vi "Process.vi"(8 "error in":errorcluster, 11 "Example Instrument UI":refnum<class "Instrument UI.PPMS.lvclass">) -> (0 "error out":errorcluster, 3 "Example Instrument UI out":refnum<class "Instrument UI.PPMS.lvclass">)   [LabVIEW 2019, in "Instrument UI.PPMS.lvclass"]
doc: "---------------------------------------------------------------\nJKI State Machine Objects™\nhttp://jki.net/state-machine-objects/\nCopyright (C) 2005-2015, JKI <info@jki.net>\nALL RIGHTS RESERVEDJKI State Machine Objects (SMO) 1.0.0.5\nJKI - JKI\nCopyright (c) 2016, JKI"
uses:
  Instrument UI.PPMS.lvclass
  <vilib>/JKI/JKI SMO/SMO/SMO.lvclass
  <vilib>/JKI/JKI SMO/SMO.UI/SMO.UI.lvclass
  <userlib>/LevyLab/Instrument Framework/Instrument/Instrument.lvclass
  instrument.PPMS/Typedefs/PPMS.getAll--cluster.ctl
  instrument.PPMS/instrument.PPMS.lvclass
  <vilib>/MakerHub/Toolbox/LMH-Toolbox.lvlib
  <userlib>/LevyLab/Instrument Framework/Instrument UI/Instrument UI.lvclass
  PPMS/PPMS.lvlib
  <userlib>/LevyLab/Configuration/Configuration.lvclass
  <userlib>/LevyLab/Instrument Framework/Instrument Types/Cryostat/Typedefs/Magnet Mode--Enum.ctl
  <userlib>/LevyLab/Instrument Framework/Instrument Types/Cryostat/Instrument.Cryostat.lvclass
  <userlib>/LevyLab/Instrument Framework/Instrument/Typedefs/Client Type--Enum.ctl
  63c30ead-59b5-487b-ba61-02a99048a75e.vi
  <userlib>/LevyLab/Instrument Framework/Instrument/API/Instrument.sendMessageToProcess (string).vi
  <userlib>/LevyLab/Debug/Debug.lvlib
  C:/Program Files (x86)/National Instruments/LabVIEW 2019/user.lib/LevyLab/Instrument Framework/Instrument UI/Instrument UI.lvclass
  C:/Program Files (x86)/National Instruments/LabVIEW 2019/vi.lib/JKI/JKI SMO/SMO.UI/SMO.UI.lvclass
  C:/Program Files (x86)/National Instruments/LabVIEW 2019/vi.lib/JKI/JKI SMO/SMO/SMO.lvclass
  C:/Program Files (x86)/National Instruments/LabVIEW 2019/user.lib/LevyLab/Instrument Framework/Instrument Types/Cryostat/Instrument.Cryostat.lvclass
  C:/Program Files (x86)/National Instruments/LabVIEW 2019/user.lib/LevyLab/Instrument Framework/Instrument/Instrument.lvclass
  instrument.PPMS/Typedefs/PPMS.Chamber Command--enum.ctl
panel:
  out "error":string="..."
  out "State":string="this is the text"
  in  "setChamber":bool
  in  "Chamber":T1="Seal"
  out "Chamber Status":string
  out "Angle (°)":dbl=90.0
  in  "setAngle":bool
  in  "Target Angle (°)":dbl format="%_3g"
  out "version":string
  out "Title":string="PPMSim"
  out "Time":dbl=90.002 format="%<%H:%M:%S %Y/%m/%d>T"
  in  "Mode":T2
  in  "B Rate (T/min)":dbl=0.1 format="%_3g"
  in  "T Rate (K/min)":dbl=300.0 format="%#_5g"
  in  "setField":bool
  in  "setTemperature":bool
  in  "Target Field (T)":dbl format="%_3g"
  in  "Target T (K)":dbl format="%#_5g"
  out "Temperature Status":string
  out "Magnet Status":string
  out "He Level (%)":dbl=90.0
  out "B (T)":dbl format="%_3f"
  out "T (K)":dbl=300.0 format="%#_5g"
  # "Local Targets"
  # "Status"
  # "SMO UI Template"
  # "For instructions on how to use the JKI State Machine Objects, examples and video tutorials, visit:\nhttp://jki.net/state-machine-objects/\n\nJKI State Machine Objects™\nhttp://jki.net/state-machine-objects/\nCopyright (C) 2005-2015, JKI <info@jki.net>\nALL RIGHTS RESERVED"
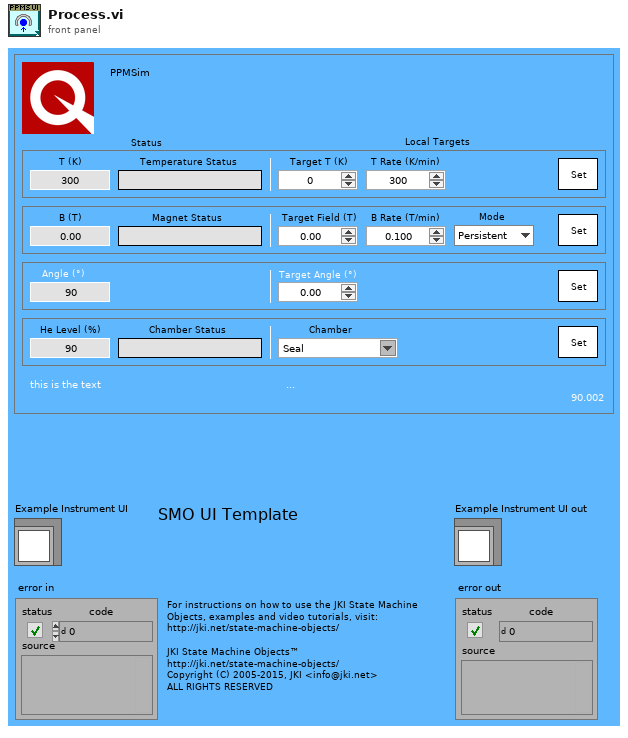
[diagram p1: front panel]
types:
  T1 = typedef "instrument.PPMS.lvclass/PPMS.Chamber Command--enum.ctl" = string
  T2 = typedef "Instrument.Cryostat.lvclass/Magnet Mode--Enum.ctl" = enum16{"Persistent", "Driven"}
  T3 = enum32{"invalid app kind", "Development System", "Run Time System", "Student Edition", "Embedded LabVIEW", "Evaluation", "Custom"}
  T4 = enum32{"Invalid", "Standard", "Closed", "Hidden", "Minimized", "Maximized"}
  T5 = typedef "instrument.PPMS.lvclass/PPMS.getAll--cluster.ctl" = cluster{"Chamber Status":string, "Helium Level":dbl, "Temperature":dbl, "Temperature Status":string, "Magnetic Field":dbl, "Magnet Status":string, "Position":dbl}
  T6 = typedef "Instrument.lvlib/Instrument.lvclass/Client Type--Enum.ctl" = enum16{"Remote", "Local"}
  T7 = typedef "PPMS.lvlib/Select PPMS--Enum.ctl" = enum16{"PPMS1", "PPMS2", "PPMS3", "PPMS-W-1", "OptiCool", "Simulate PPMS", "Simulate DynaCool", "Simulate OptiCool"}
  T8 = cluster{"Core":cluster{"Current VI Reference":refnum<vi>, "Close Panel on Exit?":bool, "Last Error":cluster{"error":errorcluster, "previous state":string, "remaining states":string}, "Shutdown?":bool}, "Instrument UI":refnum<class "Instrument UI.PPMS.lvclass">, "instrument.PPMS out":refnum<class "instrument.PPMS.lvclass">, "Data Send":variant, "Data Receive":variant, "getAll":T5, "UI Config":refnum<class "Configuration.lvclass">, "UI Cluster":cluster{"Target T (K)":dbl, "T Rate (K/min)":dbl, "Target Field (T)":dbl, "B Rate (T/min)":dbl, "Mode":T2, "Target Angle (°)":dbl}, "Client Type":T6, "Select PPMS":T7}
  T9 = cluster{"Current VI Reference":refnum<vi>, "Close Panel on Exit?":bool, "Last Error":cluster{"error":errorcluster, "previous state":string, "remaining states":string}, "Shutdown?":bool}
  T10 = cluster{"Target T (K)":dbl, "T Rate (K/min)":dbl, "Target Field (T)":dbl, "B Rate (T/min)":dbl, "Mode":T2, "Target Angle (°)":dbl}
  T11 = typedef "SMO.lvclass/Protected Events.ctl" = cluster{"StopProcesses":refnum<user-event>, "AbortProcesses":refnum<user-event>, "Config Changed":refnum<user-event>, "Dependency":refnum<user-event>}
  T12 = typedef "Instrument.lvlib/Instrument.lvclass/PublicEvents--Cluster.ctl" = cluster{"MessageFromProcess":refnum<user-event>}
  T13 = typedef "SMO.lvclass/Public Events.ctl" = cluster{"Error":refnum<user-event>, "State":refnum<user-event>, "Reserve State":refnum<user-event>}
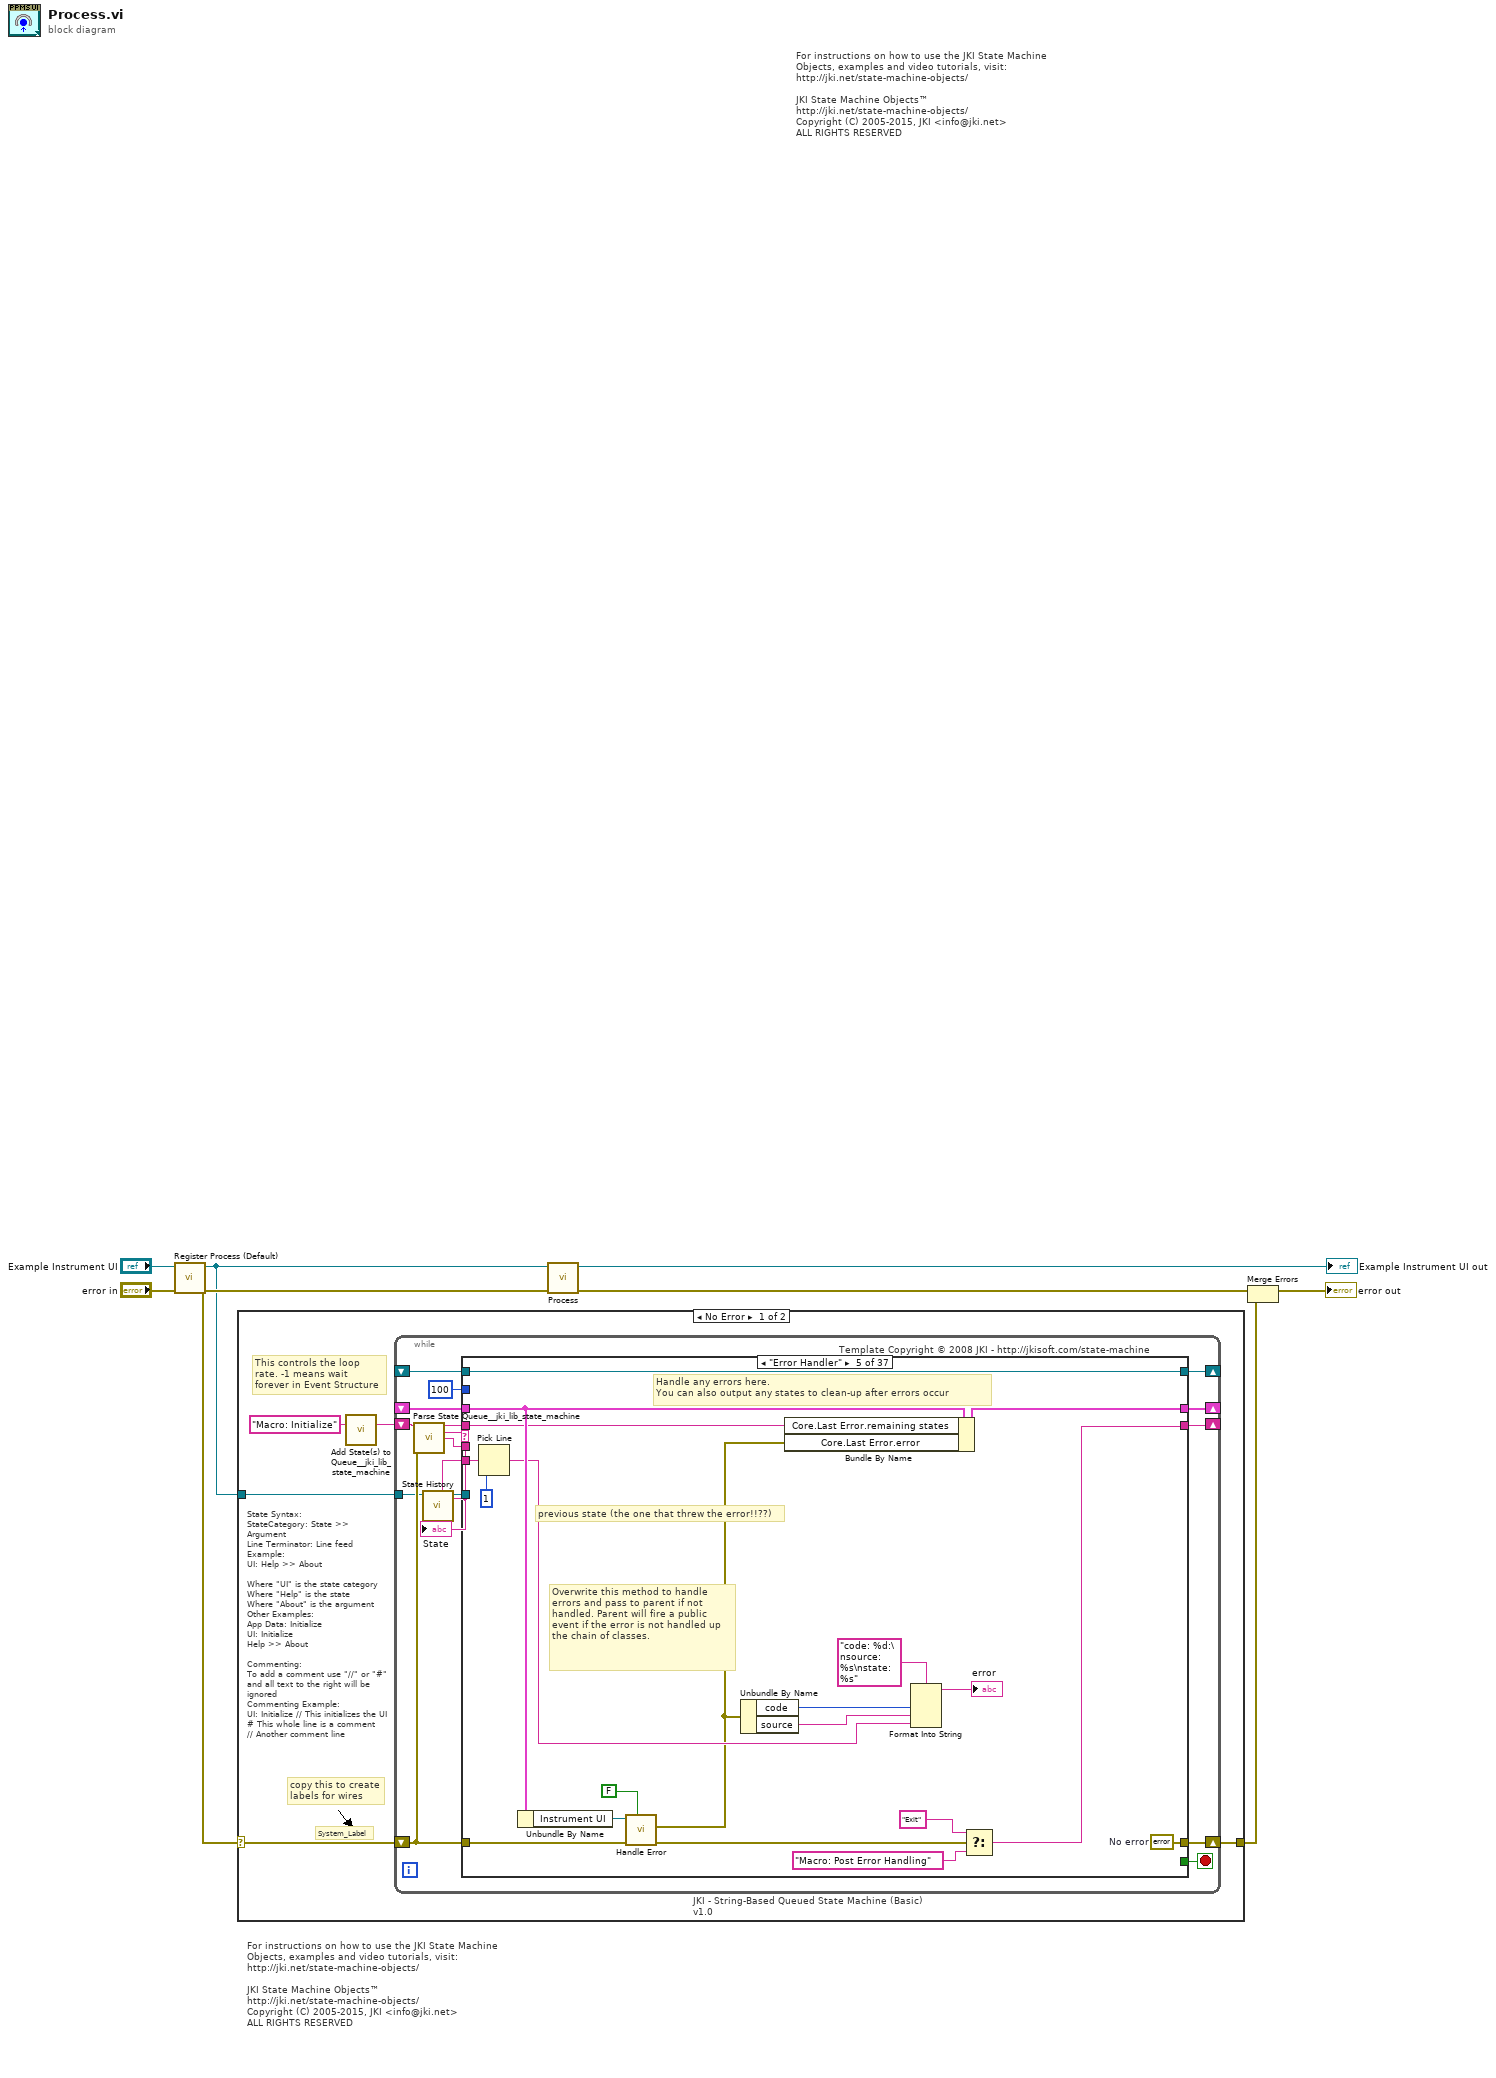
[diagram p0: block diagram]
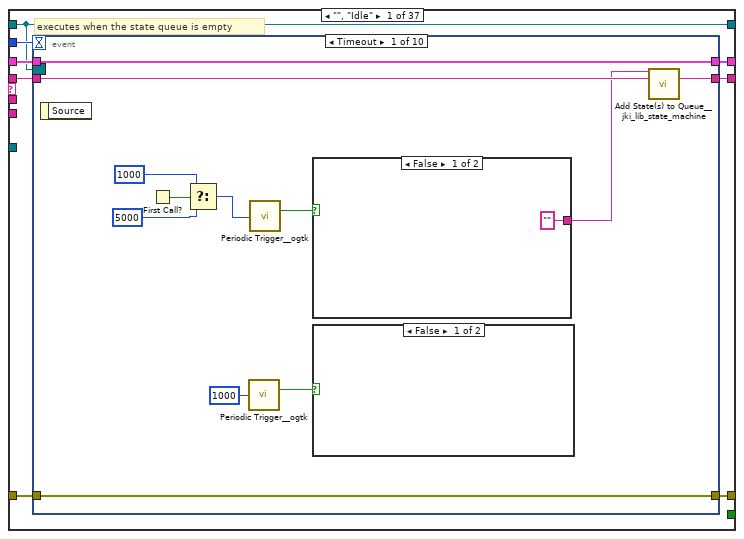
[diagram p2: hidden frame]
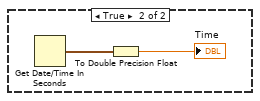
[diagram p3: hidden frame]
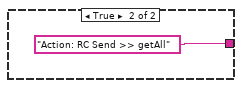
[diagram p4: hidden frame]
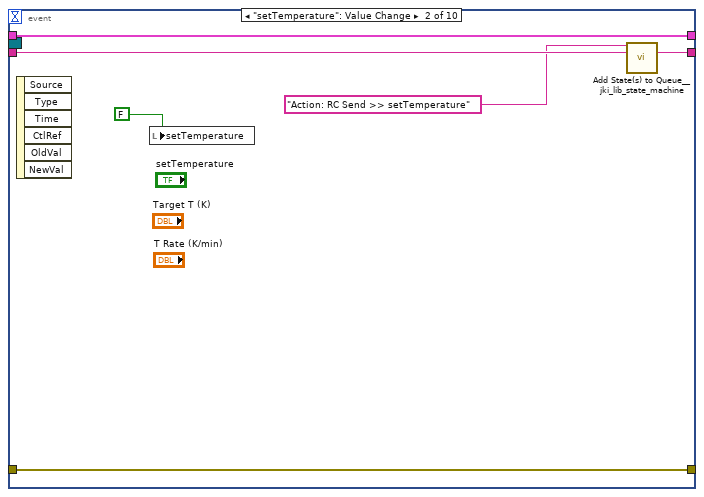
[diagram p5: hidden frame]
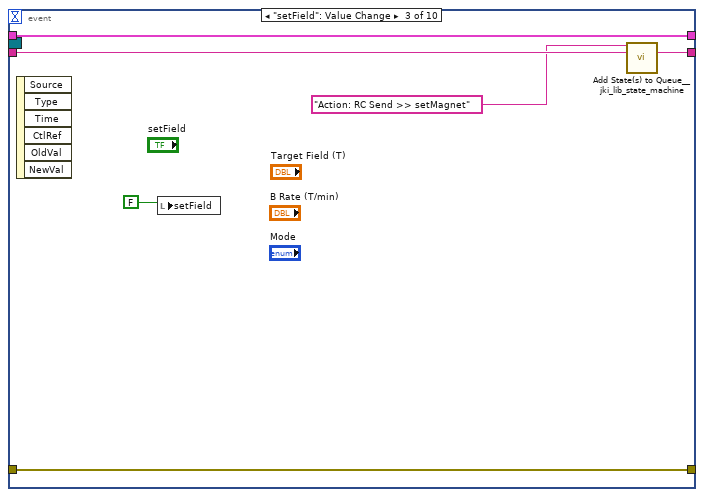
[diagram p6: hidden frame]
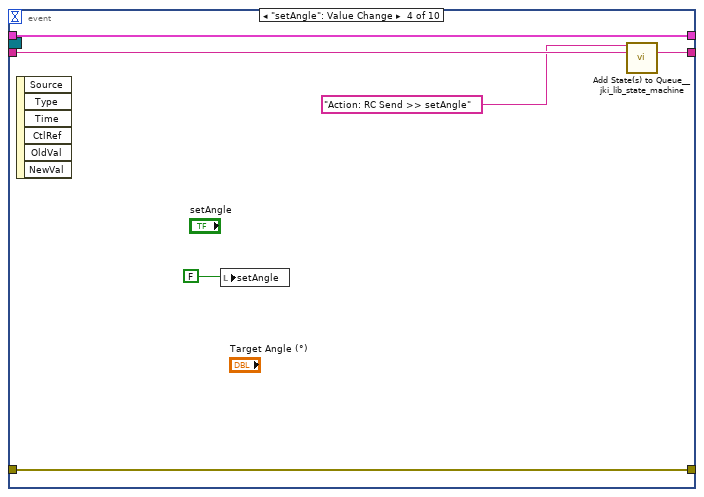
[diagram p7: hidden frame]
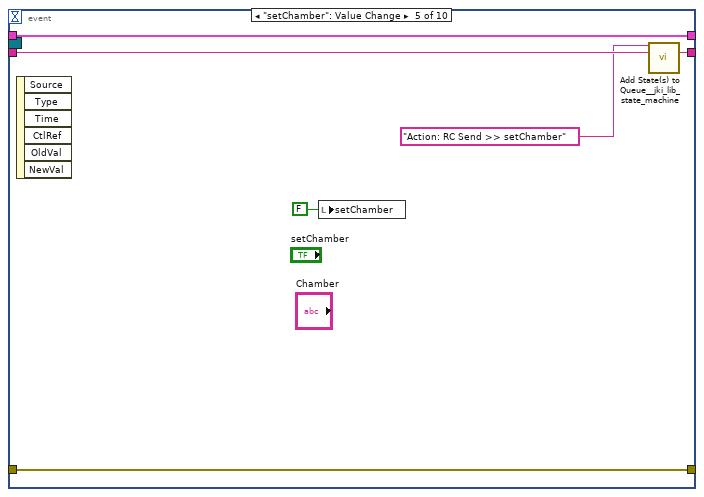
[diagram p8: hidden frame]
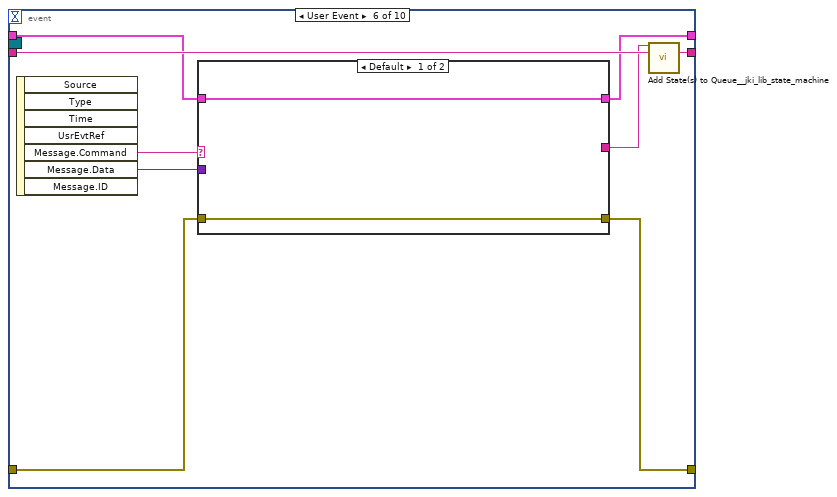
[diagram p9: hidden frame]
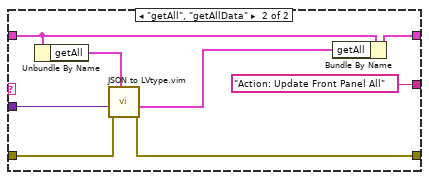
[diagram p10: hidden frame]
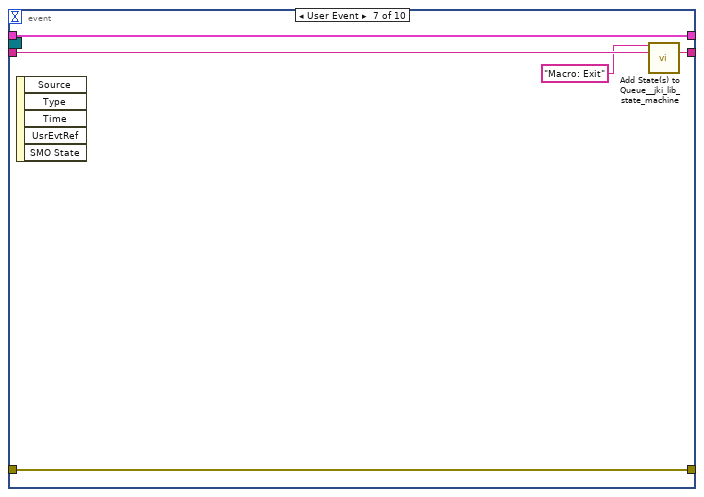
[diagram p11: hidden frame]
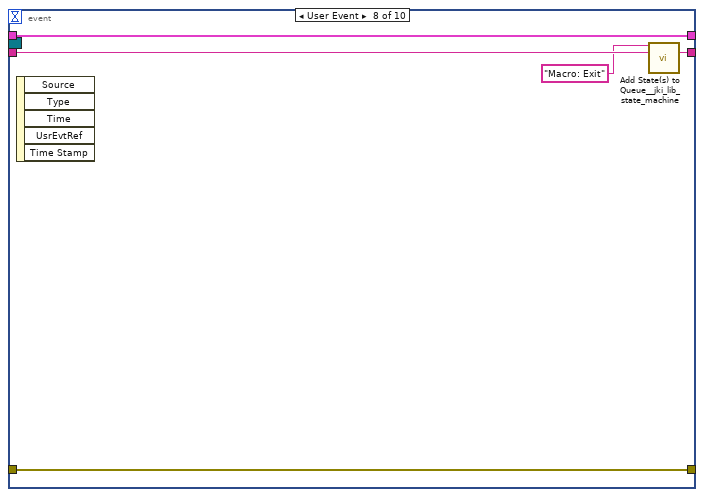
[diagram p12: hidden frame]
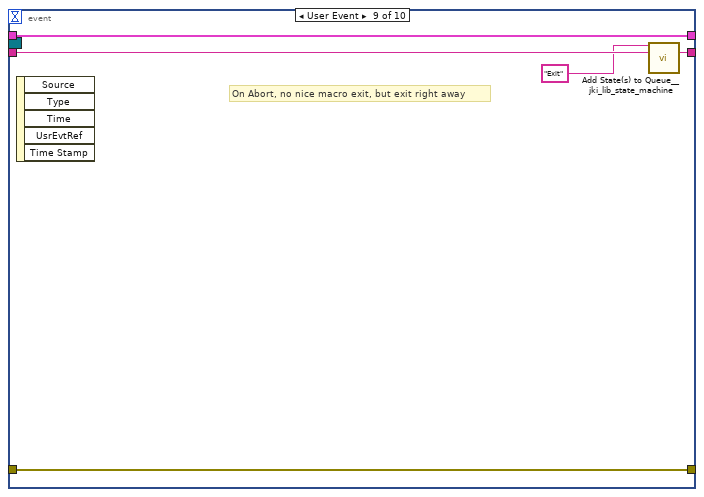
[diagram p13: hidden frame]
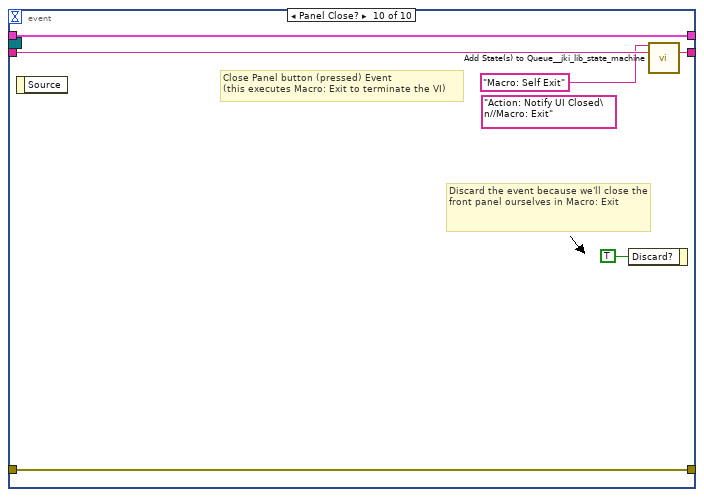
[diagram p14: hidden frame]
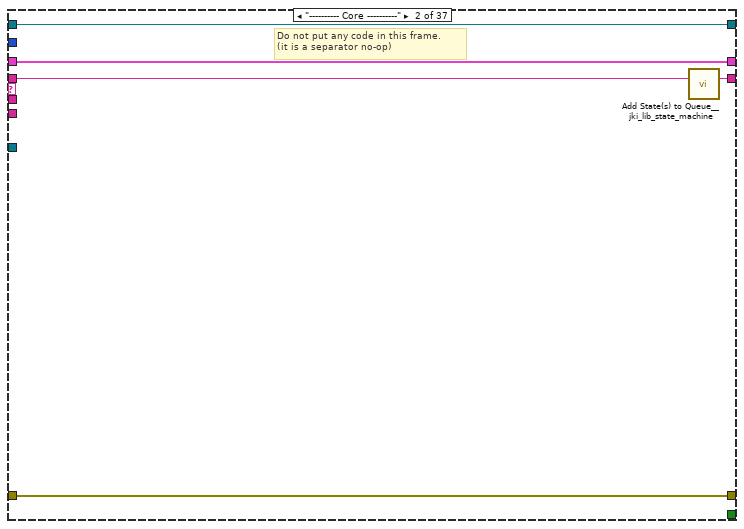
[diagram p15: hidden frame]
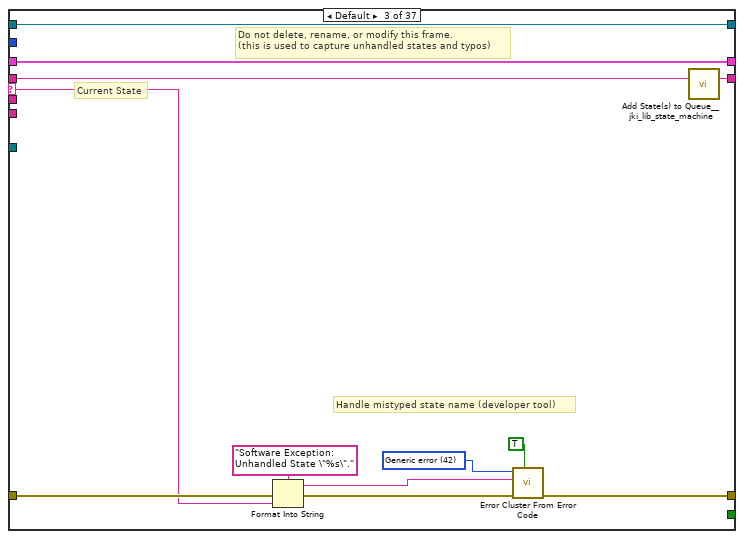
[diagram p16: hidden frame]
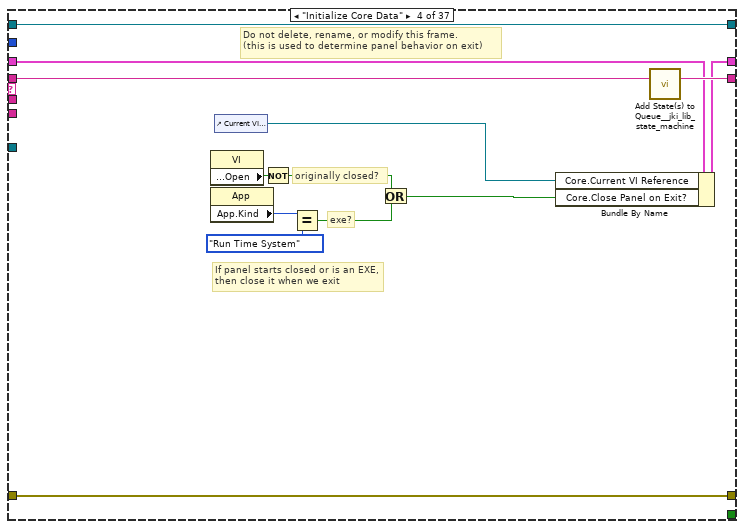
[diagram p17: hidden frame]
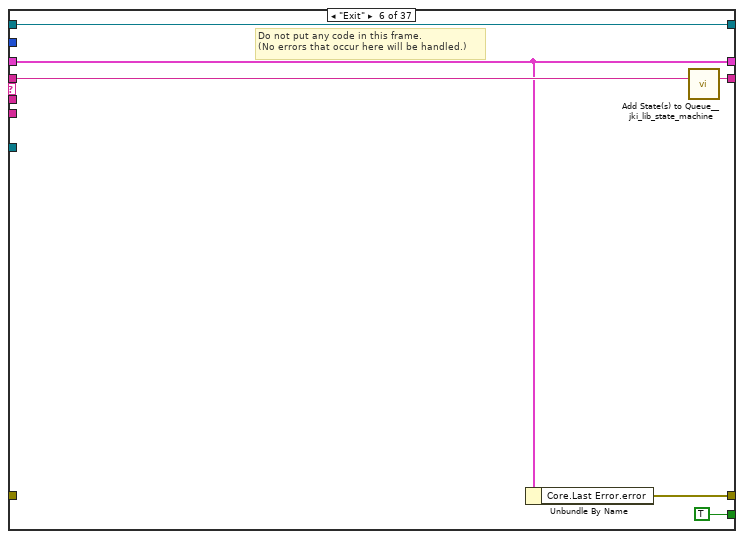
[diagram p18: hidden frame]
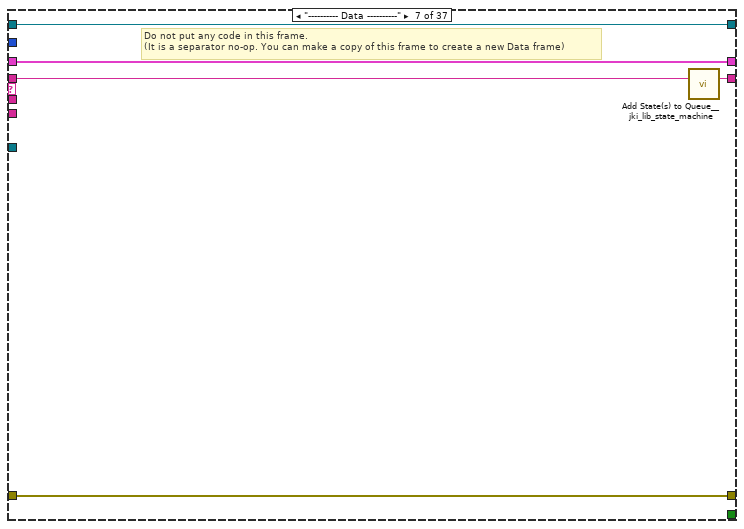
[diagram p19: hidden frame]
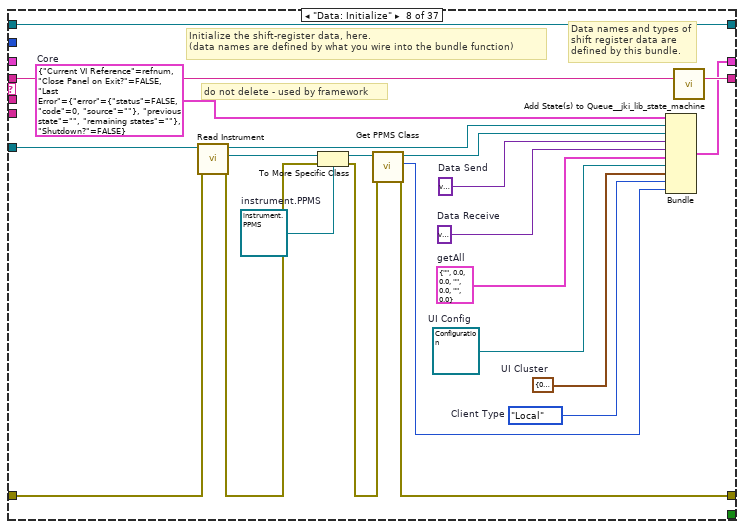
[diagram p20: hidden frame]
diagram:
  # "For instructions on how to use the JKI State Machine Objects, examples and video tutorials, visit:\nhttp://jki.net/state-machine-objects/\n\nJKI State Machine Objects™\nhttp://jki.net/state-machine-objects/\nCopyright (C) 2005-2015, JKI <info@jki.net>\nALL RIGHTS RESERVED"
  # "For instructions on how to use the JKI State Machine Objects, examples and video tutorials, visit:\nhttp://jki.net/state-machine-objects/\n\nJKI State Machine Objects™\nhttp://jki.net/state-machine-objects/\nCopyright (C) 2005-2015, JKI <info@jki.net>\nALL RIGHTS RESERVED"
  n1 = call <vilib>:"Register Process (Default).vi"("error in (no error)"="error in", "SMO"="Example Instrument UI") -> ("error out"=w5:errorcluster, "SelfRef"=w4:refnum<class "Instrument UI.PPMS.lvclass">)  [unwired: 8 in]
  n2 = case shown="No Error" w5 {
    selector: w5 -> [w10 w589]
    tunnel: w4 -> [w11 _]
    tunnel: [w9 w589] -> w1
    frame No Error {
      # "State Syntax:\nStateCategory: State >> Argument\nLine Terminator: Line feed\nExample:\nUI: Help >> About\n\nWhere \"UI\" is the state category\nWhere \"Help\" is the state\nWhere \"About\" is the argument\nOther Examples:\nApp Data: Initialize\nUI: Initialize\nHelp >> About\n\nCommenting:\nTo add a comment use \"//\" or \"#\" and all text to the right will be ignored\nCommenting Example:\nUI: Initialize // This initializes the UI\n# This whole line is a comment\n// Another comment line"
      # "copy this to create labels for wires"
      # "This controls the loop rate. -1 means wait forever in Event Structure"
      # "System_Label"
      n3 = call <vilib>:"Add State(s) to Queue__jki_lib_state_machine.vi"("State(s) in (\"\")"="Macro: Initialize") -> ("States Out"=w13:string)  [unwired: 14 in]
      n4 = while "JKI - String-Based Queued State Machine (Basic) v1.0" {
        shift-right: [w24] -> _
        shift-left: _ -> [w23]
        shift-right: [w18] -> w9
        shift-left: w10 -> [w21]
        shift-right: [w26] -> _
        shift-left: w13 -> [w27]
        tunnel: w11 -> [w16]
        shift-right: [w20] -> _
        shift-left: _ -> [w19]
        stop <- w25 stop-if-true
        # "Template Copyright © 2008 JKI - http://jkisoft.com/state-machine"
        n5 = call <vilib>:"Parse State Queue__jki_lib_state_machine.vi"("State Queue"=w27, "Error In (no error)"=w21) -> ("Remaining States"=w29:string, "Current State"=w15:string, "Arguments"=w28:string)  [unwired: 11 in]
        "State" <- w15
        n6 = call <userlib>:"State History.vi"("Current State"=w15, "SMO"=w16) -> ("SMO"=w17:refnum<class "Instrument UI.PPMS.lvclass">, "History"=w14:string)  [unwired: 8 in]
        n7 = case shown="\"Error Handler\"" w15 {
          selector: w15 -> [_ _ w124 _ _ _ _ _ _ _ _ _ _ _ _ _ _ _ _ _ _ _ _ _ _ _ _ _ _ _ _ _ _ _ _ _ _]
          tunnel: w29 -> [w37 w122 w128 w147 w149 w173 w178 w200 w208 w213 w220 w227 w243 w285 w305 w330 w354 w371 w390 w395 w404 w414 _ w446 w451 w462 w469 w476 w481 w497 w503 w510 w517 w530 w540 w547 w558]
          tunnel: w28 -> [_ _ _ _ _ _ _ _ _ _ _ w221 w237 _ _ _ _ _ _ _ _ _ _ _ _ _ _ _ _ _ _ _ _ _ _ _ w552]
          tunnel: w23 -> [w35 w119 w126 w138 w161 w169 w175 _ w205 w210 w218 w225 w239 w274 w295 w326 w350 w367 w386 w392 w400 w411 w416 w430 w448 w459 w464 w473 w478 w495 w501 w504 w511 w522 w537 w544 w548]
          tunnel: w21 -> [w33 w120 w129 w144 w162 _ w176 w184 w202 w211 w216 w223 w241 w271 w301 w324 w348 w365 w383 w393 w402 w412 w424 w444 w449 w454 w466 w472 w479 w492 w499 w507 w513 w524 w531 w541 w553]
          tunnel: [w36 w121 w127 w146 w150 w172 w177 w199 w207 w212 w219 w226 w242 w284 w304 w329 w353 w370 w389 w394 w403 w413 w425 w445 w450 w461 w468 w475 w480 w496 w502 w509 w516 w529 w539 w546 w557] -> w26
          tunnel: [_ _ _ _ _ TRUE _ _ _ _ _ _ _ _ _ _ _ _ _ _ _ _ _ _ _ _ _ _ _ _ _ _ _ _ _ _ _] -> w25
          tunnel: [w32 w119 w126 w145 w164 w169 w175 w198 w205 w210 w218 w225 w239 w275 w296 w327 w351 w368 w387 w392 w400 w411 w417 w431 w448 w459 w464 w473 w478 w495 w501 w506 w511 w522 w536 w543 w549] -> w24
          tunnel: 100 ("Timeout") -> [w31 _ _ _ _ _ _ _ _ _ _ _ _ _ _ _ _ _ _ _ _ _ _ _ _ _ _ _ _ _ _ _ _ _ _ _ _]
          tunnel: w17 -> [_ _ _ _ _ _ _ w186 _ _ _ _ _ _ _ _ _ _ _ _ _ _ _ _ _ _ _ _ _ _ _ _ _ _ _ _ _]
          tunnel: [w30 w118 w123 w135 w167 w170 w174 w197 w204 w209 w217 w224 w236 w283 w303 w328 w352 w369 w388 w391 w401 w410 w423 w438 w447 w460 w467 w474 w477 w494 w500 w508 w515 w528 w538 w545 w556] -> w20
          tunnel: w19 -> [w30 w118 w123 w135 w167 w170 w174 w197 w204 w209 w217 w224 w236 w283 w303 w328 w352 w369 w388 w391 w401 w410 w423 w438 w447 w460 w467 w474 w477 _ w500 w508 w515 w528 w538 w545 w556]
          tunnel: [w34 w120 w130 w144 w165 w168 w176 w179 w206 w211 w215 w222 w240 w271 w301 w324 w342 w364 w382 w393 w402 w412 w424 w444 w449 w453 w465 w471 w479 w490 w498 w507 w512 w524 w532 w541 w554] -> w18
          tunnel: w14 -> [_ _ _ _ w155 _ _ _ _ _ _ _ _ _ _ _ _ _ _ _ _ _ _ _ _ _ _ _ _ _ _ _ _ _ _ _ _]
          frame "", "Idle" {
            # "executes when the state queue is empty"
            n8 = event shown="[0] Timeout" {
              selector: w30 -> [_ _ _ _ _ _ _ _ _ _]
              dyn-events: _ -> [_ _ _ _ _ _ _ _ _ _]
              timeout: w31 -> [_ _ _ _ _ _ _ _ _ _]
              tunnel: w37 -> [w49 w56 w62 w68 w77 w86 w101 w106 w111 w117]
              tunnel: [w48 w58 w64 w70 w76 w85 w100 w105 w110 w116] -> w36
              tunnel: w35 -> [w46 w57 w63 w69 w74 w80 w98 w103 w108 w114]
              tunnel: [w47 w59 w65 w71 w75 w78 w99 w104 w109 w113] -> w34
              tunnel: w33 -> [w47 w59 w65 w71 w75 w79 w99 w104 w109 w113]
              tunnel: [w46 w57 w63 w69 w74 w81 w98 w103 w108 w114] -> w32
              event Timeout {
                n9 = event-data() -> ()  [unwired: 1 in, 1 out]
                n10 = First Call?() -> (First Call?: T/F=w41:bool)
                n11 = Select(t=u32 1000 ("update time (ms)"), s=w41, f=u32 5000 ("update time (ms)")) -> (s? t:f=w38:u32)
                n12 = call <userlib>:"Periodic Trigger__ogtk.vi"("time (ms)"=u32 1000) -> ("Triggered"=w42:bool)  [unwired: 12 in, 2 out]
                n13 = call <userlib>:"Periodic Trigger__ogtk.vi"("time (ms)"=w38) -> ("Triggered"=w45:bool)  [unwired: 12 in, 2 out]
                n14 = case shown="False" w45 {
                  tunnel: ["" "Action: RC Send >> getAll"] -> w44
                  frame False {
                  }
                  frame True {
                  }
                }
                n15 = case shown="False" w42 {
                  frame False {
                  }
                  frame True {
                    n16 = Get Date/Time In Seconds() -> (seconds since 1Jan1904=w51:timestamp)
                    n17 = To Double Precision Float(number=w51) -> (double precision float=→"Time":dbl)
                  }
                }
                n18 = call <vilib>:"Add State(s) to Queue__jki_lib_state_machine.vi"("State(s) in Front (\"\")"=w44, "State(s) in (\"\")"=w49) -> ("States Out"=w48:string)  [unwired: 13 in]
              }
              event "setTemperature": Value Change {
                n19 = event-data() -> ()  [unwired: 1 in, 6 out]
                n20 = local write "setTemperature"(FALSE ("Temperature")) -> ()
                n21 = call <vilib>:"Add State(s) to Queue__jki_lib_state_machine.vi"("State(s) in Front (\"\")"="Action: RC Send >> setTemperature" ("State(s) in Front (\"\")"), "State(s) in (\"\")"=w56) -> ("States Out"=w58:string)  [unwired: 13 in]
              }
              event "setField": Value Change {
                n22 = event-data() -> ()  [unwired: 1 in, 6 out]
                n23 = local write "setField"(FALSE ("Field")) -> ()
                n24 = call <vilib>:"Add State(s) to Queue__jki_lib_state_machine.vi"("State(s) in Front (\"\")"="Action: RC Send >> setMagnet" ("State(s) in Front (\"\")"), "State(s) in (\"\")"=w62) -> ("States Out"=w64:string)  [unwired: 13 in]
              }
              event "setAngle": Value Change {
                n25 = event-data() -> ()  [unwired: 1 in, 6 out]
                n26 = local write "setAngle"(FALSE ("Angle")) -> ()
                n27 = call <vilib>:"Add State(s) to Queue__jki_lib_state_machine.vi"("State(s) in Front (\"\")"="Action: RC Send >> setAngle" ("State(s) in Front (\"\")"), "State(s) in (\"\")"=w68) -> ("States Out"=w70:string)  [unwired: 13 in]
              }
              event "setChamber": Value Change {
                n28 = event-data() -> ()  [unwired: 1 in, 6 out]
                n29 = local write "setChamber"(FALSE ("Set Chamber")) -> ()
                n30 = call <vilib>:"Add State(s) to Queue__jki_lib_state_machine.vi"("State(s) in Front (\"\")"="Action: RC Send >> setChamber" ("State(s) in Front (\"\")"), "State(s) in (\"\")"=w77) -> ("States Out"=w76:string)  [unwired: 13 in]
              }
              event User Event {
                n31 = event-data() -> ("Message.Command"=w83:string, "Message.Data"=w82:variant)  [unwired: 1 in, 5 out]
                n32 = case shown="Default" w83 {
                  tunnel: [_ "Action: Update Front Panel All" ("State(s) in Front (\"\")")] -> w84
                  tunnel: w82 -> [_ w94]
                  tunnel: w80 -> [w88 w89]
                  tunnel: [w88 w95] -> w81
                  tunnel: w79 -> [w87 w90]
                  tunnel: [w87 w91] -> w78
                  frame Default {
                  }
                  frame "getAll", "getAllData" {
                    n33 = Unbundle By Name(w89) -> ("getAll"=w93:T5)
                    n34 = call "JSON to LVtype.vim"("type"=w93, "error in (no error)"=w90, "JSON Data in"=w94) -> ("error out"=w91:errorcluster, "Data out"=w92:T5)  [unwired: 7 in]
                    n35 = Bundle By Name(cluster=w89, "getAll"=w92) -> (w95:T8)
                  }
                }
                n36 = call <vilib>:"Add State(s) to Queue__jki_lib_state_machine.vi"("State(s) in Front (\"\")"=w84, "State(s) in (\"\")"=w86) -> ("States Out"=w85:string)  [unwired: 13 in]
              }
              event User Event {
                n37 = event-data() -> ()  [unwired: 1 in, 5 out]
                n38 = call <vilib>:"Add State(s) to Queue__jki_lib_state_machine.vi"("State(s) in Front (\"\")"="Macro: Exit", "State(s) in (\"\")"=w101) -> ("States Out"=w100:string)  [unwired: 13 in]
              }
              event User Event {
                n39 = event-data() -> ()  [unwired: 1 in, 5 out]
                n40 = call <vilib>:"Add State(s) to Queue__jki_lib_state_machine.vi"("State(s) in Front (\"\")"="Macro: Exit", "State(s) in (\"\")"=w106) -> ("States Out"=w105:string)  [unwired: 13 in]
              }
              event User Event {
                # "On Abort, no nice macro exit, but exit right away"
                n41 = event-data() -> ()  [unwired: 1 in, 5 out]
                n42 = call <vilib>:"Add State(s) to Queue__jki_lib_state_machine.vi"("State(s) in Front (\"\")"="Exit", "State(s) in (\"\")"=w111) -> ("States Out"=w110:string)  [unwired: 13 in]
              }
              event Panel Close? {
                (unwired) "Action: Notify UI Closed\n//Macro: Exit"
                # "Discard the event because we'll close the front panel ourselves in Macro: Exit"
                # "Close Panel button (pressed) Event\n(this executes Macro: Exit to terminate the VI)"
                n43 = event-data() -> ()  [unwired: 1 in, 1 out]
                n44 = event-data("Discard?"=TRUE) -> ()  [unwired: 1 in, 1 out]
                n45 = call <vilib>:"Add State(s) to Queue__jki_lib_state_machine.vi"("State(s) in Front (\"\")"="Macro: Self Exit" ("State(s) in Front (\"\")"), "State(s) in (\"\")"=w117) -> ("States Out"=w116:string)  [unwired: 13 in]
              }
            }
          }
          frame "---------- Core ----------" {
            # "Do not put any code in this frame.\n(it is a separator no-op)"
            n46 = call <vilib>:"Add State(s) to Queue__jki_lib_state_machine.vi"("State(s) in (\"\")"=w122) -> ("States Out"=w121:string)  [unwired: 14 in]
          }
          frame Default {
            w133 = 42 items=["No error", "Argument error", "Memory is full", "Out of zone", "End of file", "File already open", "Generic file I/O error", "File not found", "File permission error", "Disk is full", "Duplicate path", "Too many files open", "System feature not enabled", "Resource file not found", "Cannot add resource", "Resource not found", "Image not found", "Image memory error", "Pen does not exist", "Config type invalid", "Config token not found", "Config parse error", "Config memory error", "Bad external code format", "Bad external code offset", "External code not present", "Null window", "Destroy window error", "Null menu", "Print aborted", "Bad print record", "Print driver error", "Windows error during printing", "Memory error during printing", "Print dialog error", "Generic print error", "Invalid device refnum", "Device not found", "Device parameter error", "Device unit error", "Cannot open device", "Device call aborted", "Generic error", "Cancelled by user", "Object ID too low", "Object ID too high", "Object not in heap", "Unknown heap", "Unknown object (invalid DefProc)", "Unknown object (DefProc not in table)", "Message out of range", "Invalid (null) method", "Unknown message", "Manager call not supported", "Bad address", "Network operation in progress", "Network operation timed out", "Connection is busy", "Network attribute not supported", "Network error", "Address in use", "System out of memory", "Connection aborted", "Connection refused", "Not connected", "Already connected", "Connection closed", "Initialization error (interapplication manager)", "Bad occurrence", "Wait on unbound occurrence handler", "Occurrence queue overflow", "Datalog type conflict", "Unused", "Unrecognized type (interapplication manager)", "Memory corrupt", "Failed to make temporary DLL", "Old CIN version", "Drag socket not found", "Failed to load drop-object", "Failed to register OLE object", "Failed to release OLE object", "Format specifier type mismatch", "Unknown format specifier", "Too few format specifiers", "Too many format specifiers", "Scan failed", "Newer CIN version", "Error converting to variant", "Runtime menu error", "Password tampered", "Variant attribute not found", "Incompatible variant data type", "Event data is not available", "Event Store is not present", "Occurrence is not found", "Event Queue is not created", "Event info is not available", "Refnum passed is NULL", "Error retrieving Class GUID", "Error retrieving CoClass GUID", "Error retrieving TypeLib GUID.", "Bad built application magic bytes.", "Specific driver is different from the specific driver associated with the Logical Name.", "There is no session opened to the class driver.", "Max Error", "MAX - Error with config objects", "MAX - Error loading configuration", "MAX - Group not supported"]
            # "Current State"
            # "Do not delete, rename, or modify this frame.\n(this is used to capture unhandled states and typos)"
            # "Handle mistyped state name (developer tool)"
            n47 = Format Into String(format string="Software Exception: Unhandled State \"%s\"." ("message"), error in=w129, w124) -> (resulting string=w132:string, error out=w131:errorcluster)  [unwired: 1 in]
            n48 = call <vilib>:"Error Cluster From Error Code.vi"("show call chain? (False)"=TRUE, "error in (no error)"=w131, "error message (\"\")"=w132, "error code (0)"=w133) -> ("error out"=w130:errorcluster)  [unwired: 5 in]
            n49 = call <vilib>:"Add State(s) to Queue__jki_lib_state_machine.vi"("State(s) in (\"\")"=w128) -> ("States Out"=w127:string)  [unwired: 14 in]
          }
          frame "Initialize Core Data" {
            # "Do not delete, rename, or modify this frame.\n(this is used to determine panel behavior on exit)"
            # "originally closed?"
            # "exe?"
            # "If panel starts closed or is an EXE, then close it when we exit"
            n50 = property class="VI"() -> ("Front Panel.Open"=w143:bool)  [unwired: 2 in, 2 out]
            n51 = property class="App"() -> ("App.Kind"=w142:T3)  [unwired: 2 in, 2 out]
            n52 = control-ref of="Current VI Reference"() -> (w136:refnum<vi>)
            n53 = Not(x=w143) -> (.not. x?=w140:bool)
            n54 = Equal?(x=w142, y=T3."Run Time System" ("Application:Kind")) -> (x = y?=w139:bool)
            n55 = Or(x=w140, y=w139) -> (x .or. y?=w137:bool)
            n56 = Bundle By Name(cluster=w138, "Core.Current VI Reference"=w136, "Core.Close Panel on Exit?"=w137) -> (w145:T8)
            n57 = call <vilib>:"Add State(s) to Queue__jki_lib_state_machine.vi"("State(s) in (\"\")"=w147) -> ("States Out"=w146:string)  [unwired: 14 in]
          }
          frame "Error Handler" {
            w165 = errorcluster {"status"=FALSE, "code"=0, "source"=""}  # No error
            # "previous state (the one that threw the error!!??)"
            # "Overwrite this method to handle errors and pass to parent if not handled. Parent will fire a public event if the error is not handled up the chain of classes."
            # "Handle any errors here.\nYou can also output any states to clean-up after errors occur"
            n58 = Pick Line(multi-line string=w155, line index=1) -> (output string=w153:string)  [unwired: 1 in]
            n59 = Unbundle By Name(w161) -> ("Instrument UI"=w166:refnum<class "Instrument UI.PPMS.lvclass">)
            n60 = call-dynamic "Handle Error.vi"("Stop on Unhandled Error (T)"=FALSE, "error in"=w162, "SMO"=w166) -> ("handling error"=w160:errorcluster, "Unhandled error"=w148:errorcluster)  [unwired: 6 in, 1 out]
            n61 = Unbundle By Name(w148) -> ("code"=w157:i32, "source"=w156:string)
            n62 = Bundle By Name(cluster=w161, "Core.Last Error.remaining states"=w149, "Core.Last Error.error"=w148) -> (w164:T8)
            n63 = Format Into String(format string="code: %d:\nsource: %s\nstate: %s", w157, w156, w153) -> (resulting string=→"error":string)  [unwired: 2 in, 1 out]
            n64 = Select(t="Exit", s=w160, f="Macro: Post Error Handling") -> (s? t:f=w150:string)
          }
          frame "Exit" {
            # "Do not put any code in this frame.\n(No errors that occur here will be handled.)"
            n65 = Unbundle By Name(w169) -> ("Core.Last Error.error"=w168:errorcluster)
            n66 = call <vilib>:"Add State(s) to Queue__jki_lib_state_machine.vi"("State(s) in (\"\")"=w173) -> ("States Out"=w172:string)  [unwired: 14 in]
          }
          frame "---------- Data ----------" {
            # "Do not put any code in this frame.\n(It is a separator no-op. You can make a copy of this frame to create a new Data frame)"
            n67 = call <vilib>:"Add State(s) to Queue__jki_lib_state_machine.vi"("State(s) in (\"\")"=w178) -> ("States Out"=w177:string)  [unwired: 14 in]
          }
          frame "Data: Initialize" {
            w185 = T9 {"Current VI Reference"=refnum, "Close Panel on Exit?"=FALSE, "Last Error"={"error"={"status"=FALSE, "code"=0, "source"=""}, "previous state"="", "remaining states"=""}, "Shutdown?"=FALSE}  # Core
            w187 = Client_Type--Enum."Local"  # Client Type
            w188 = T10 {"Target T (K)"=0.0, "T Rate (K/min)"=0.0, "Target Field (T)"=0.0, "B Rate (T/min)"=0.0, "Mode"=enum."Persistent", "Target Angle (°)"=0.0}  # UI Cluster
            w189 = refnum<class "Configuration.lvclass"> refnum  # UI Config
            w190 = refnum<class "instrument.PPMS.lvclass"> refnum  # instrument.PPMS
            w194 = T5 {"Chamber Status"="", "Helium Level"=0.0, "Temperature"=0.0, "Temperature Status"="", "Magnetic Field"=0.0, "Magnet Status"="", "Position"=0.0}  # getAll
            w195 = variant  # Data Receive
            w196 = variant  # Data Send
            # "do not delete - used by framework"
            # "Data names and types of shift register data are defined by this bundle."
            # "Initialize the shift-register data, here.\n(data names are defined by what you wire into the bundle function)"
            n68 = call <userlib>:"Read Instrument.vi"("error in (no error)"=w184, "Instrument UI in"=w186) -> ("error out"=w193:errorcluster, "Instrument"=w191:refnum<class "Instrument.lvclass">, "Instrument UI"=w192:refnum<class "Instrument UI.PPMS.lvclass">)  [unwired: 7 in]
            n69 = To More Specific Class(target class=w190, reference=w191, error in=w193) -> (specific class reference=w182:refnum<class "instrument.PPMS.lvclass">, error out=w180:errorcluster)
            n70 = call "Get PPMS Class.vi"("error in (no error)"=w180, "instrument.PPMS"=w182) -> ("error out"=w179:errorcluster, "Select PPMS"=w183:T7, "instrument.PPMS out"=w181:refnum<class "instrument.PPMS.lvclass">)  [unwired: 7 in]
            n71 = Bundle("Core"=w185, "Instrument UI"=w192, "instrument.PPMS out"=w181, "Data Send"=w196, "Data Receive"=w195, "getAll"=w194, "UI Config"=w189, "UI Cluster"=w188, "Client Type"=w187, "Select PPMS"=w183) -> (w198:T8)  [unwired: 1 in]
            n72 = call <vilib>:"Add State(s) to Queue__jki_lib_state_machine.vi"("State(s) in (\"\")"=w200) -> ("States Out"=w199:string)  [unwired: 14 in]
          }
          frame "Data: Cleanup" {
            # "Cleanup any data and references, here.\n(this is called automatically, by the Macro: Exit)"
            n73 = Unbundle By Name(w205) -> ("Core.Current VI Reference"=w203:refnum<vi>)
            n74 = call <vilib>:"Save State As Default.vi"("Error In"=w202, "Target VI"=w203) -> ("Error Out"=w201:errorcluster)  [unwired: 8 in, 1 out]
            n75 = Close Reference(reference=w203, error in (no error)=w201) -> (error out=w206:errorcluster)
            n76 = call <vilib>:"Add State(s) to Queue__jki_lib_state_machine.vi"("State(s) in (\"\")"=w208) -> ("States Out"=w207:string)  [unwired: 14 in]
          }
          frame "---------- UI ----------" {
            # "Do not put any code in this frame.\n(It is a separator no-op. You can make a copy of this frame to create a new UI frame)"
            n77 = call <vilib>:"Add State(s) to Queue__jki_lib_state_machine.vi"("State(s) in (\"\")"=w213) -> ("States Out"=w212:string)  [unwired: 14 in]
          }
          frame "UI: Initialize" {
            # "size window to decoration box on front panel"
            # "Initialize the User Interface, here.\n(this is called automatically, by the Macro: Init)"
            n78 = call <userlib>:"Fit VI window to Largest Dec__ogtk.vi"("error in (no error)"=w216, "border spacing (2 px)"=0) -> ("error out"=w215:errorcluster)  [unwired: 4 in, 1 out]
            n79 = call <vilib>:"Add State(s) to Queue__jki_lib_state_machine.vi"("State(s) in (\"\")"=w220) -> ("States Out"=w219:string)  [unwired: 14 in]
          }
          frame "UI: Cursor Set" {
            # "Argument"
            # "Initialize the User Interface, here.\n(this is called automatically, by the Macro: Init)"
            n80 = disable-structure shown="Default" {
              disable-tunnel: w223 -> [w228 w231]
              disable-tunnel: [w228 w230] -> w222
              disable-tunnel: w221 -> [_ w229]
              frame condition #0 {
              }
              frame condition #1 (active) {
                n81 = case shown="\"Idle\", Default" w229 {
                  tunnel: w231 -> [w233 w235]
                  tunnel: [w232 w234] -> w230
                  frame "Idle", Default {
                    n82 = call <vilib>:"Unset Busy.vi"("error in (no error)"=w233) -> ("error out"=w232:errorcluster)  [unwired: 10 in]
                  }
                  frame "Busy" {
                    n83 = call <vilib>:"Set Busy.vi"("error in (no error)"=w235) -> ("error out"=w234:errorcluster)  [unwired: 9 in, 1 out]
                  }
                }
              }
            }
            n84 = call <vilib>:"Add State(s) to Queue__jki_lib_state_machine.vi"("State(s) in (\"\")"=w227) -> ("States Out"=w226:string)  [unwired: 14 in]
          }
          frame "UI: Front Panel State" {
            # "Argument"
            # "Set Front Panel Open or Closed\n(Usage: \"UI: Front Panel State >> Open|Close\")"
            n85 = Unbundle By Name(w239) -> ("Core.Current VI Reference"=w238:refnum<vi>)
            n86 = disable-structure shown="Default" {
              disable-tunnel: w241 -> [w247 w270]
              disable-tunnel: [w246 w270] -> w240
              disable-tunnel: w238 -> [w245 _]
              disable-tunnel: w237 -> [w244 _]
              frame condition #0 (active) {
                n87 = case shown="\"Close\"" w244 {
                  tunnel: w247 -> [w251 w264]
                  tunnel: [w253 w265] -> w246
                  tunnel: w245 -> [w252 w262]
                  frame "Open", Default {
                    n88 = property class="VI"(reference=w252, error in=w251) -> (reference out=w249:refnum<vi>, error out=w250:errorcluster, "FP.State"=w248:T4)
                    n89 = case shown="\"Closed\"" w248 {
                      tunnel: [w256 w259] -> w253
                      tunnel: w250 -> [w255 w259]
                      tunnel: w249 -> [w254 _]
                      frame "Closed" {
                        n90 = invoke class="VI" method="FP.Open"(reference=w254, error in=w255, "Activate"=TRUE, "State"=T4."Standard") -> (error out=w256:errorcluster)  [unwired: 1 in, 4 out]
                      }
                      frame Default {
                      }
                    }
                  }
                  frame "Close" {
                    n91 = property class="VI"(reference=w262, error in=w264) -> (reference out=w261:refnum<vi>, error out=w263:errorcluster, "FP.State"=w260:T4)
                    n92 = case shown="Default" w260 {
                      tunnel: [w266 w269] -> w265
                      tunnel: w263 -> [w266 w268]
                      tunnel: w261 -> [_ w267]
                      frame "Invalid", "Closed" {
                      }
                      frame Default {
                        n93 = invoke class="VI" method="FP.Close"(reference=w267, error in=w268) -> (error out=w269:errorcluster)  [unwired: 1 in, 2 out]
                      }
                    }
                  }
                }
              }
              frame condition #1 {
              }
            }
            n94 = call <vilib>:"Add State(s) to Queue__jki_lib_state_machine.vi"("State(s) in (\"\")"=w243) -> ("States Out"=w242:string)  [unwired: 14 in]
          }
          frame "UI: Set Background Color" {
            n95 = Unbundle By Name(w274) -> ("instrument.PPMS out"=w272:refnum<class "instrument.PPMS.lvclass">, "Select PPMS"=w273:T7)
            n96 = property class="VI"() -> (error out=w281:errorcluster, "Panel"=w280:refnum<vi>)  [unwired: 2 in, 1 out]
            n97 = case shown="\"OptiCool\"" w273 {
              tunnel: [u32 9077092 ("Color Box") u32 32639 ("Color Box") u32 6273022 ("Color Box") u32 14592465 ("Color Box") u32 16763690 ("Color Box") u32 16758979 ("Color Box") u32 12369084 ("Color Box") u32 16762248 ("Color Box")] -> w276
              frame "PPMS1", Default {
              }
              frame "PPMS2" {
              }
              frame "PPMS3" {
              }
              frame "PPMS-W-1" {
              }
              frame "OptiCool" {
              }
              frame "Simulate PPMS" {
              }
              frame "Simulate DynaCool" {
              }
              frame "Simulate OptiCool" {
              }
            }
            n98 = property class="Pnl"(reference=w280, error in=w281) -> (error out=w282:errorcluster, "Panes[]"=w279:refnum<vi>[])  [unwired: 1 out]
            n99 = Index Array(array=w279, index=0) -> (element=w277:refnum<vi>)
            n100 = Bundle By Name(cluster=w274, "instrument.PPMS out"=w272) -> (w275:T8)
            n101 = property class="Pane"(reference=w277, error in=w282, "PaneColor"=w276) -> ()  [unwired: 2 out]
            n102 = call <vilib>:"Add State(s) to Queue__jki_lib_state_machine.vi"("State(s) in (\"\")"=w285) -> ("States Out"=w284:string)  [unwired: 14 in]
          }
          frame "UI: Set Title" {
            n103 = Unbundle By Name(w295) -> ("instrument.PPMS out"=w297:refnum<class "instrument.PPMS.lvclass">, "Select PPMS"=w294:T7)
            n104 = case shown="\"Simulate PPMS\"..\"Simulate OptiCool\"" w294 {
              selector: w294 -> [w307 w309]
              tunnel: [w306 w310] -> w302
              frame "Simulate PPMS".."Simulate OptiCool" {
                n105 = Format Into String(format string="%s", w307) -> (resulting string=w306:string)  [unwired: 2 in, 1 out]
              }
              frame Default {
                n106 = Format Into String(format string="%s Monitor and Control" ("Title"), w309) -> (resulting string=w310:string)  [unwired: 2 in, 1 out]
              }
            }
            "Title" <- w302
            n107 = call <userlib>:"MGI Get Executable Version.vi"() -> ("Version"=w299:string)  [unwired: 7 in]
            n108 = Concatenate Strings("v" ("string"), w299) -> (→"version":string)
            n109 = Bundle By Name(cluster=w295, "instrument.PPMS out"=w297) -> (w296:T8)
            n110 = call <vilib>:"Add State(s) to Queue__jki_lib_state_machine.vi"("State(s) in (\"\")"=w305) -> ("States Out"=w304:string)  [unwired: 14 in]
          }
          frame "UI: Hide Controls" {
            # "OptiCool: Hide He Level and Chamber control\nand PPMS-W-1 (DynaCool)"
            # "Only show rotator control for PPMS2 and PPMS3"
            # "UI: Hide Controls\n(It is a separator no-op. You can make a copy of this frame to create a new UI frame)"
            n111 = Unbundle By Name(w326) -> ("instrument.PPMS out"=w325:refnum<class "instrument.PPMS.lvclass">, "Select PPMS"=w313:T7)
            n112 = case shown="\"Simulate DynaCool\"" w313 {
              tunnel: [TRUE ("Visible") FALSE ("Visible") FALSE ("Visible") FALSE ("Visible")] -> w314
              frame Default {
              }
              frame "OptiCool", "Simulate OptiCool" {
              }
              frame "Simulate DynaCool" {
              }
              frame "PPMS-W-1" {
              }
            }
            n113 = case shown="\"PPMS2\"" w313 {
              tunnel: [FALSE ("Visible") TRUE ("Visible")] -> w319
              frame Default {
              }
              frame "PPMS2" {
              }
            }
            n114 = control-ref of="setAngle"() -> (w323:refnum<vi>)
            n115 = control-ref of="Chamber"() -> (w316:refnum<vi>)
            n116 = control-ref of="Target Angle (°)"() -> (w322:refnum<vi>)
            n117 = control-ref of="Angle (°)"() -> (w321:refnum<vi>)
            n118 = control-ref of="setChamber"() -> (w315:refnum<vi>)
            n119 = control-ref of="He Level (%)"() -> (w318:refnum<vi>)
            n120 = control-ref of="Mode"() -> (w312:refnum<vi>)
            n121 = Build Array(w323, w322, w321) -> (w320:refnum<vi>[])
            n122 = Build Array(w318, w316, w315, w312) -> (w317:refnum<vi>[])
            n123 = Bundle By Name(cluster=w326, "instrument.PPMS out"=w325) -> (w327:T8)
            n124 = for {
              tunnel: w317 -> [w332] mode=indexing
              tunnel: w314 -> [w331]
              n125 = property class="Ctl"(reference=w332, "Visible"=w331) -> ()  [unwired: 1 in, 2 out]
            }
            n126 = for {
              tunnel: w320 -> [w334] mode=indexing
              tunnel: w319 -> [w333]
              n127 = property class="Ctl"(reference=w334, "Visible"=w333) -> ()  [unwired: 1 in, 2 out]
            }
            n128 = call <vilib>:"Add State(s) to Queue__jki_lib_state_machine.vi"("State(s) in (\"\")"=w330) -> ("States Out"=w329:string)  [unwired: 14 in]
          }
          frame "UI: Init UI Config" {
            # "Do not put any code in this frame.\n(It is a separator no-op. You can make a copy of this frame to create a new UI frame)"
            n129 = Unbundle By Name(w350) -> ("instrument.PPMS out"=w341:refnum<class "instrument.PPMS.lvclass">)
            n130 = call <vilib>:"GetName.vi"("error in (no error)"=w348, "SMO"=w341) -> ("error out"=w347:errorcluster, "Name"=w349:string)  [unwired: 6 in, 2 out]
            n131 = call <userlib>:"Default Path.vi"("error in (no error)"=w347, "Folder Name [Application Name]"=w349) -> ("error out"=w343:errorcluster, "Configuration out"=w346:refnum<class "Configuration.lvclass">)  [unwired: 8 in]
            n132 = call <userlib>:"Write Section.vi"("error in (no error)"=w343, "Section"="UI", "Configuration in"=w346) -> ("error out"=w342:errorcluster, "Configuration out"=w344:refnum<class "Configuration.lvclass">)  [unwired: 7 in]
            n133 = Bundle By Name(cluster=w350, "instrument.PPMS out"=w341, "UI Config"=w344) -> (w351:T8)
            n134 = call <vilib>:"Add State(s) to Queue__jki_lib_state_machine.vi"("State(s) in (\"\")"=w354) -> ("States Out"=w353:string)  [unwired: 14 in]
          }
          frame "UI: Write UI Config" {
            # "Do not put any code in this frame.\n(It is a separator no-op. You can make a copy of this frame to create a new UI frame)"
            n135 = local read "Target Angle (°)"() -> (w357:dbl)
            n136 = local read "Target Field (T)"() -> (w360:dbl)
            n137 = local read "T Rate (K/min)"() -> (w361:dbl)
            n138 = local read "B Rate (T/min)"() -> (w359:dbl)
            n139 = Unbundle By Name(w367) -> ("UI Config"=w366:refnum<class "Configuration.lvclass">, "UI Cluster"=w356:T10)
            n140 = local read "Target T (K)"() -> (w362:dbl)
            n141 = local read "Mode"() -> (w358:T2)
            n142 = Bundle By Name(cluster=w356, "Target T (K)"=w362, "T Rate (K/min)"=w361, "Target Field (T)"=w360, "B Rate (T/min)"=w359, "Mode"=w358, "Target Angle (°)"=w357) -> (w355:T10)
            n143 = call <userlib>:"Write Configuration.vi"("error in (no error)"=w365, "Variant"=w355, "Configuration in"=w366) -> ("error out"=w364:errorcluster, "Configuration out"=w363:refnum<class "Configuration.lvclass">)  [unwired: 7 in]
            n144 = Bundle By Name(cluster=w367, "UI Config"=w363) -> (w368:T8)
            n145 = call <vilib>:"Add State(s) to Queue__jki_lib_state_machine.vi"("State(s) in (\"\")"=w371) -> ("States Out"=w370:string)  [unwired: 14 in]
          }
          frame "UI: Read UI Config" {
            # "Do not put any code in this frame.\n(It is a separator no-op. You can make a copy of this frame to create a new UI frame)"
            n146 = Unbundle By Name(w386) -> ("UI Cluster"=w379:T10, "UI Config"=w384:refnum<class "Configuration.lvclass">)
            n147 = call <userlib>:"Read Configuration.vi"("INI Fomatted Cluster Type"=w379, "error in (no error)"=w383, "Configuration in"=w384) -> ("error out"=w385:errorcluster, "Configuration"=w381:variant, "Configuration out"=w380:refnum<class "Configuration.lvclass">)  [unwired: 6 in]
            n148 = Variant To Data(error in=w385, type=w379, Variant=w381) -> (data=w378:T10, error out=w382:errorcluster)
            n149 = Unbundle By Name(w378) -> ("Target T (K)"=w377:dbl, "T Rate (K/min)"=w376:dbl, "Target Field (T)"=w375:dbl, "B Rate (T/min)"=w374:dbl, "Mode"=w373:T2, "Target Angle (°)"=w372:dbl)
            n150 = local write "Target T (K)"(w377) -> ()
            n151 = local write "T Rate (K/min)"(w376) -> ()
            n152 = local write "Target Field (T)"(w375) -> ()
            n153 = local write "B Rate (T/min)"(w374) -> ()
            n154 = local write "Mode"(w373) -> ()
            n155 = local write "Target Angle (°)"(w372) -> ()
            n156 = Bundle By Name(cluster=w386, "UI Config"=w380) -> (w387:T8)
            n157 = call <vilib>:"Add State(s) to Queue__jki_lib_state_machine.vi"("State(s) in (\"\")"=w390) -> ("States Out"=w389:string)  [unwired: 14 in]
          }
          frame "---------- Macro ----------" {
            # "Do not put any code in this frame.\n(It is a separator no-op. You can make a copy of this frame to create a new Macro frame)"
            n158 = call <vilib>:"Add State(s) to Queue__jki_lib_state_machine.vi"("State(s) in (\"\")"=w395) -> ("States Out"=w394:string)  [unwired: 14 in]
          }
          frame "Macro: Initialize" {
            # "Initialization Macro\n(This is called once, when the VI starts)"
            n159 = call <vilib>:"Add State(s) to Queue__jki_lib_state_machine.vi"("State(s) in Front (\"\")"="Data: Initialize\nInitialize Core Data\nEvents: Register", "State(s) in (\"\")"="Process: Sync", "State(s) at Back (\"\")"="UI: Initialize\nUI: Front Panel State >> Open\nUI: Set Background Color\nUI: Set Title\nUI: Hide Controls\nUI: Init UI Config\nUI: Read UI Config\nAction: Open") -> ("States Out"=w397:string)  [unwired: 12 in]
            n160 = call <vilib>:"Add State(s) to Queue__jki_lib_state_machine.vi"("State(s) in Front (\"\")"=w397, "State(s) in (\"\")"=w404) -> ("States Out"=w403:string)  [unwired: 13 in]
          }
          frame "Macro: Self Exit" {
            (unwired) "Action: Notify UI Closed\nMacro: Exit"
            n161 = Two Button Dialog(message="Are you sure you want to stop this program?") -> (T button?=w409:bool)  [unwired: 2 in]
            n162 = Select(t="//Process: Stop Instrument\nUI: Front Panel State >> Close\nProcess: Self Terminate\nMacro: Exit", s=w409, f="") -> (s? t:f=w405:string)
            n163 = call <vilib>:"Add State(s) to Queue__jki_lib_state_machine.vi"("State(s) in Front (\"\")"=w405, "State(s) in (\"\")"=w414) -> ("States Out"=w413:string)  [unwired: 13 in]
          }
          frame "Macro: Post Error Handling" {
            # "Clear Last Error?"
            n164 = Unbundle By Name(w416) -> ("Core.Last Error.remaining states"=w418:string, "Core.Shutdown?"=w419:bool)
            n165 = Unbundle By Name(w416) -> ("Core.Last Error.error"=w422:errorcluster)
            n166 = case shown="False" FALSE {
              tunnel: w422 -> [w429 _]
              tunnel: [w429 _] -> w421
              frame False {
              }
              frame True {
              }
            }
            n167 = case shown="False" w419 {
              tunnel: w418 -> [_ w428]
              tunnel: ["Action: Close\nAction: Open\n" ("State(s) in Front (\"\")") w427] -> w415
              frame False {
                # "These are the remaining states (at the moment the error occured). States can be altered according to business logic."
                # "NOT SHUTTING DOWN"
              }
              frame True {
                # "Developer can decide to alter the states but should be aware that during the shutdown process, there are certain states that must be run for the SMO to properly shut itself (and this process) down. As such, one can add states to perform additional clean-ups, but should append the remaining state to be executed."
                # "SHUTTING DOWN"
                n168 = call <vilib>:"Add State(s) to Queue__jki_lib_state_machine.vi"("State(s) in (\"\")"=w428) -> ("States Out"=w427:string)  [unwired: 14 in]
              }
            }
            n169 = Bundle By Name(cluster=w416, "Core.Last Error.error"=w421) -> (w417:T8)
            n170 = call <vilib>:"Add State(s) to Queue__jki_lib_state_machine.vi"("State(s) in Front (\"\")"=w415) -> ("States Out"=w425:string)  [unwired: 14 in]
          }
          frame "Macro: Exit" {
            # "Exit Macro\n(This is called once, when the VI exits)"
            n171 = Unbundle By Name(w430) -> ("Core.Close Panel on Exit?"=w443:bool)
            n172 = Bundle By Name(cluster=w430, "Core.Shutdown?"=TRUE) -> (w431:T8)
            n173 = Select(t="UI: Front Panel State >> Close", s=w443, f="") -> (s? t:f=w440:string)
            n174 = call <vilib>:"Add State(s) to Queue__jki_lib_state_machine.vi"("State(s) in Front (\"\")"="Data: Cleanup\nEvents: Unregister", "State(s) in (\"\")"="Process: Sync", "State(s) at Back (\"\")"="Exit") -> ("States Out"=w435:string)  [unwired: 12 in]
            n175 = call <vilib>:"Add State(s) to Queue__jki_lib_state_machine.vi"("State(s) in Front (\"\")"="Action: Close\nUI: Write UI Config", "State(s) in (\"\")"=w440, "State(s) at Back (\"\")"=w435) -> ("States Out"=w439:string)  [unwired: 12 in]
            n176 = call <vilib>:"Add State(s) to Queue__jki_lib_state_machine.vi"("State(s) in Front (\"\")"=w439, "State(s) in (\"\")"=w446) -> ("States Out"=w445:string)  [unwired: 13 in]
          }
          frame "---------- Process ----------" {
            # "Template Separator\n(You can make a copy of, or modify, this frame)"
            n177 = call <vilib>:"Add State(s) to Queue__jki_lib_state_machine.vi"("State(s) in (\"\")"=w451) -> ("States Out"=w450:string)  [unwired: 14 in]
          }
          frame "Process: Sync" {
            n178 = Unbundle By Name(w459) -> ("Instrument UI"=w455:refnum<class "Instrument UI.PPMS.lvclass">)
            n179 = call <vilib>:"WaitOnProcessSync.vi"("error in (no error)"=w454, "SMO"=w455) -> ("error out"=w453:errorcluster, "Don't run?"=w458:bool)  [unwired: 7 in, 1 out]
            n180 = Select(t="Data: Cleanup\nEvents: Unregister\nExit", s=w458, f="") -> (s? t:f=w452:string)
            n181 = call <vilib>:"Add State(s) to Queue__jki_lib_state_machine.vi"("State(s) in Front (\"\")"=w452, "State(s) in (\"\")"=w462) -> ("States Out"=w461:string)  [unwired: 13 in]
          }
          frame "Process: Self Terminate" {
            n182 = Unbundle By Name(w464) -> ("Instrument UI"=w463:refnum<class "Instrument UI.PPMS.lvclass">)
            n183 = call <vilib>:"SelfTerminate.vi"("error in (no error)"=w466, "SMO in"=w463) -> ("error out"=w465:errorcluster)  [unwired: 8 in, 1 out]
            n184 = call <vilib>:"Add State(s) to Queue__jki_lib_state_machine.vi"("State(s) in (\"\")"=w469) -> ("States Out"=w468:string)  [unwired: 14 in]
          }
          frame "Process: Stop Instrument" {
            # "Template Separator\n(You can make a copy of, or modify, this frame)"
            n185 = Unbundle By Name(w473) -> ("instrument.PPMS out"=w470:refnum<class "instrument.PPMS.lvclass">)
            n186 = call <vilib>:"Stop.vi"("error in (no error)"=w472, "SMO"=w470) -> ("error out"=w471:errorcluster)  [unwired: 8 in, 1 out]
            n187 = call <vilib>:"Add State(s) to Queue__jki_lib_state_machine.vi"("State(s) in (\"\")"=w476) -> ("States Out"=w475:string)  [unwired: 14 in]
          }
          frame "---------- Events ----------" {
            # "Template Separator\n(You can make a copy of, or modify, this frame)"
            n188 = call <vilib>:"Add State(s) to Queue__jki_lib_state_machine.vi"("State(s) in (\"\")"=w481) -> ("States Out"=w480:string)  [unwired: 14 in]
          }
          frame "Events: Register" {
            # "Expand to add\nmore events"
            # "Base Class Protected Events"
            n189 = Unbundle By Name(w495) -> ("Instrument UI"=w488:refnum<class "Instrument UI.PPMS.lvclass">, "instrument.PPMS out"=w482:refnum<class "instrument.PPMS.lvclass">)
            n190 = call <vilib>:"GetProtectedEvents.vi"("SMO"=w488) -> ("error out"=w489:errorcluster, "SMO Protected Events"=w493:T11)  [unwired: 8 in, 1 out]
            n191 = call <userlib>:"Instrument.GetPublicEvents.vi"("Instrument"=w482) -> ("error out"=w486:errorcluster, "Instrument Public Events"=w487:T12, "Instrument out"=w485:refnum<class "instrument.PPMS.lvclass">)  [unwired: 8 in]
            n192 = call <vilib>:"GetPublicEvents.vi"("SMO"=w485) -> ("error out"=w483:errorcluster, "Public Events"=w484:T13)  [unwired: 8 in, 1 out]
            n193 = register-events(w493, w487, w484) -> (reference out=w494:refnum<event-registration>, error out=w491:errorcluster)  [unwired: 2 in]
            n194 = Merge Errors(w483, w486, w492, w491, w489) -> (w490:errorcluster)
            n195 = call <vilib>:"Add State(s) to Queue__jki_lib_state_machine.vi"("State(s) in (\"\")"=w497) -> ("States Out"=w496:string)  [unwired: 14 in]
          }
          frame "Events: Unregister" {
            n196 = Unregister For Events(event registration refnum=w500, error in=w499) -> (error out=w498:errorcluster)
            n197 = call <vilib>:"Add State(s) to Queue__jki_lib_state_machine.vi"("State(s) in (\"\")"=w503) -> ("States Out"=w502:string)  [unwired: 14 in]
          }
          frame "---------- Action ----------" {
            n198 = Unbundle By Name(w504) -> ("Instrument UI"=w505:refnum<class "Instrument UI.PPMS.lvclass">)
            n199 = Bundle By Name(cluster=w504, "Instrument UI"=w505) -> (w506:T8)
            n200 = call <vilib>:"Add State(s) to Queue__jki_lib_state_machine.vi"("State(s) in (\"\")"=w510) -> ("States Out"=w509:string)  [unwired: 14 in]
          }
          frame "Action: Notify UI Closed" {
            # "Notify that the UI has been closed"
            n201 = Unbundle By Name(w511) -> ("Instrument UI"=w514:refnum<class "Instrument UI.PPMS.lvclass">)
            n202 = call <vilib>:"Hide.vi"("error in (no error)"=w513, "SMO.UI"=w514) -> ("error out"=w512:errorcluster)  [unwired: 8 in, 1 out]
            n203 = call <vilib>:"Add State(s) to Queue__jki_lib_state_machine.vi"("State(s) in (\"\")"=w517) -> ("States Out"=w516:string)  [unwired: 14 in]
          }
          frame "Action: Update Front Panel All" {
            n204 = Unbundle By Name(w522) -> ("getAll"=w525:T5)
            n205 = Unbundle By Name(w525) -> ("Helium Level"=→"He Level (%)":dbl, "Temperature"=→"T (K)":dbl, "Temperature Status"=→"Temperature Status":string, "Magnetic Field"=→"B (T)":dbl, "Magnet Status"=→"Magnet Status":string, "Position"=→"Angle (°)":dbl, "Chamber Status"=→"Chamber Status":string)
            n206 = call <vilib>:"Add State(s) to Queue__jki_lib_state_machine.vi"("State(s) in (\"\")"=w530) -> ("States Out"=w529:string)  [unwired: 14 in]
          }
          frame "Action: Open" {
            n207 = Unbundle By Name(w537) -> ("instrument.PPMS out"=w535:refnum<class "instrument.PPMS.lvclass">, "Client Type"=w533:T6)
            n208 = call <userlib>:"Write Client Type.vi"("error in (no error)"=w531, "Client Type [Remote]"=w533, "Instrument in"=w535) -> ("error out"=w532:errorcluster, "Instrument out"=w534:refnum<class "instrument.PPMS.lvclass">)  [unwired: 7 in]
            n209 = Bundle By Name(cluster=w537, "instrument.PPMS out"=w534) -> (w536:T8)
            n210 = call <vilib>:"Add State(s) to Queue__jki_lib_state_machine.vi"("State(s) in (\"\")"=w540) -> ("States Out"=w539:string)  [unwired: 14 in]
          }
          frame "Action: Close" {
            n211 = Unbundle By Name(w544) -> ("instrument.PPMS out"=w542:refnum<class "instrument.PPMS.lvclass">)
            n212 = Bundle By Name(cluster=w544, "instrument.PPMS out"=w542) -> (w543:T8)
            n213 = call <vilib>:"Add State(s) to Queue__jki_lib_state_machine.vi"("State(s) in (\"\")"=w547) -> ("States Out"=w546:string)  [unwired: 14 in]
          }
          frame "Action: RC Send" {
            (unwired) ""
            n214 = Unbundle By Name(w548) -> ("instrument.PPMS out"=w555:refnum<class "instrument.PPMS.lvclass">, "Data Send"=w551:variant)
            n215 = case shown="\"setMagnet\"" w552 {
              tunnel: w555 -> [w560 w563 w570 w576 w579 w588]
              tunnel: [w559 w561 w569 w574 w578 w586] -> w554
              tunnel: w553 -> [w559 w562 w568 w575 w577 w587]
              tunnel: w551 -> [_ _ _ _ _ _]
              tunnel: [w560 w564 w571 w573 w580 w585] -> w550
              frame Default {
              }
              frame "getAll", "getAllData" {
                n216 = call-poly <userlib>:"Instrument.sendMessageToProcess.vi"("error in (no error)"=w562, "Command"="getAllData", "Instrument"=w563) -> ("error out"=w561:errorcluster, "Instrument out"=w564:refnum<class "instrument.PPMS.lvclass">)  [unwired: 7 in]
              }
              frame "setTemperature" {
                n217 = local read "T Rate (K/min)"() -> (w566:dbl)
                n218 = local read "Target T (K)"() -> (w567:dbl)
                n219 = call-dynamic "setTemperature.vi"("error in (no error)"=w568, "Rate (K/min)"=w566, "Temperature (K)"=w567, "instrument.PPMS"=w570) -> ("error out"=w569:errorcluster, "instrument.PPMS out"=w571:refnum<class "instrument.PPMS.lvclass">)  [unwired: 6 in]
              }
              frame "setAngle" {
                n220 = local read "Target Angle (°)"() -> (w572:dbl)
                n221 = call-dynamic "setAngle.vi"("error in (no error)"=w575, "Angle (°)"=w572, "instrument.PPMS"=w576) -> ("error out"=w574:errorcluster, "instrument.PPMS out"=w573:refnum<class "instrument.PPMS.lvclass">)  [unwired: 7 in]
              }
              frame "setMagnet" {
                n222 = local read "Target Field (T)"() -> (w583:dbl)
                n223 = local read "B Rate (T/min)"() -> (w582:dbl)
                n224 = local read "Mode"() -> (w581:T2)
                n225 = call-dynamic "setMagnet.vi"("Mode"=w581, "error in (no error)"=w577, "Target Rate (T/min)"=w582, "Target Field (T)"=w583, "instrument.PPMS"=w579) -> ("error out"=w578:errorcluster, "instrument.PPMS out"=w580:refnum<class "instrument.PPMS.lvclass">)  [unwired: 5 in]
              }
              frame "setChamber" {
                n226 = local read "Chamber"() -> (w584:T1)
                n227 = call-dynamic "setChamber.vi"("error in (no error)"=w587, "Action"=w584, "instrument.PPMS in"=w588) -> ("error out"=w586:errorcluster, "instrument.PPMS out"=w585:refnum<class "instrument.PPMS.lvclass">)  [unwired: 7 in]
              }
            }
            n228 = Bundle By Name(cluster=w548, "instrument.PPMS out"=w550) -> (w549:T8)
            n229 = call <vilib>:"Add State(s) to Queue__jki_lib_state_machine.vi"("State(s) in (\"\")"=w558) -> ("States Out"=w557:string)  [unwired: 14 in]
          }
        }
      }
    }
    frame Error {
    }
  }
  n230 = call-parent "Process.vi"("error in"=w5, "Instrument UI in"=w4) -> ("error out"=w2:errorcluster, "Instrument UI out"=→"Example Instrument UI out":refnum<class "Instrument UI.PPMS.lvclass">)  [unwired: 8 in]
  n231 = Merge Errors(w2, w1) -> (→"error out":errorcluster)
